vi "Save Max Value (SubVI).vi"(11 "value in":dbl) -> (3 "value out":dbl)   [LabVIEW 2020]
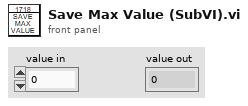
[diagram p1: front panel]
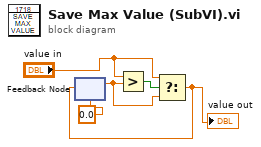
[diagram p0: block diagram]
diagram:
  n1 = feedback #1(0.0 ("acceleration")) -> (w2:dbl)
  n2 = Greater?(x="value in", y=w2) -> (0:w4:bool)
  n3 = Select(t="value in", s=w4, f=w2) -> (s? t:f=w1:dbl)
  "value out" <- w1
  n4 = feedback-in #1(w1) -> ()
